vi "SaveDataQRef.vi"(8 "error in (no error)":errorcluster, 11 "Interface.lvclass":refnum<class "Interface.lvclass">) -> (0 "error out":errorcluster, 3 "Interface.lvclass Out":refnum<class "Interface.lvclass">)   [LabVIEW 2019, in "Interface.lvclass"]
uses:
  Interface.lvclass
  Interface.lvclass/Interface.ctl
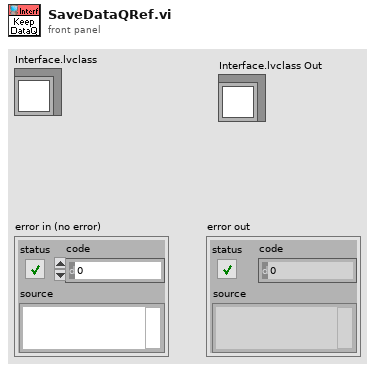
[diagram p1: front panel]
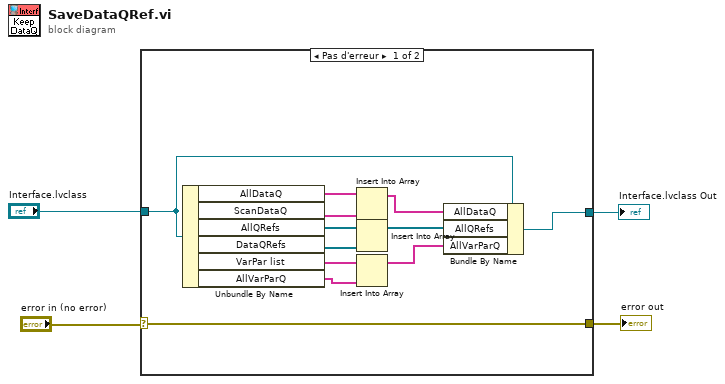
[diagram p0: block diagram]
diagram:
  n1 = case shown="Pas d'erreur" "error in (no error)" {
    selector: "error in (no error)" -> [w16 w18]
    tunnel: [w16 w18] -> w3
    tunnel: "Interface.lvclass" -> [w15 w17]
    tunnel: [w11 w17] -> w1
    frame No Error {
      n2 = Unbundle By Name(w15) -> ("AllDataQ"=w14:string[], "ScanDataQ"=w13:string[], "AllQRefs"=w10:refnum<queue>[], "DataQRefs"=w9:refnum<queue>[], "VarPar list"=w7:string[], "AllVarParQ"=w6:string[])
      n3 = Insert Into Array(array=w14, new element=w13) -> (w12:string[])  [unwired: 1 in]
      n4 = Insert Into Array(array=w10, new element=w9) -> (w8:refnum<queue>[])  [unwired: 1 in]
      n5 = Insert Into Array(array=w7, new element=w6) -> (w5:string[])  [unwired: 1 in]
      n6 = Bundle By Name(cluster=w15, "AllDataQ"=w12, "AllQRefs"=w8, "AllVarParQ"=w5) -> (w11:refnum<class "Interface.lvclass">)
    }
    frame Error {
    }
  }
  "error out" <- w3
  "Interface.lvclass Out" <- w1
